vi "CAPTH-Init IPC.vi"() -> (8 "IPC":T1)   [LabVIEW 2020]
uses:
  Typedefs/CAPTH-IPC.ctl
  Typedefs/CAPTH-Start Data.ctl
  Typedefs/CAPTH-Parameters.ctl
  Typedefs/CAPTH-Stimulus.ctl
  Typedefs/CAPTH-Response.ctl
  Typedefs/CAPTH-Analysis Message.ctl
  Typedefs/CAPTH-Analysis Action.ctl
  Typedefs/CAPTH-StimCon.ctl
  Typedefs/CAPTH-Analysis Data Properties.ctl
panel:
  out "queue out":refnum<queue>
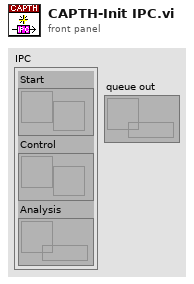
[diagram p1: front panel]
types:
  T1 = typedef "CAPTH-IPC.ctl" = cluster{"Start":refnum<notifier>, "Control":refnum<notifier>, "Analysis":refnum<queue>}
  T2 = typedef "CAPTH-Analysis Message.ctl" = cluster{"Action":T3, "Data":dbl[], "StimCon":T4, "Properties":T5, "Num":i32}
  T3 = typedef "CAPTH-Analysis Action.ctl" = enum16{"Init", "Raw", "Avg", "Quit"}
  T4 = typedef "CAPTH-StimCon.ctl" = cluster{"ear":i32, "freq":i32, "Max SPL":dbl}
  T5 = typedef "CAPTH-Analysis Data Properties.ctl" = cluster{"atten":dbl, "amp":dbl, "1dB":bool}
  T6 = typedef "CAPTH-Start Data.ctl" = cluster{"Datafile":path, "Params":T7, "data":cluster{"Freq":dbl[], "Threshold atten":dbl[], "Max SPL":dbl[]}[]}
  T7 = typedef "CAPTH-Parameters.ctl" = cluster{"Stimulus":T8, "Response":T9}
  T8 = typedef "CAPTH-Stimulus.ctl" = cluster{"EAR":enum16{"RIGHT", "LEFT\n", "ALTERNATE"}, "HI FREQ":dbl, "LO FREQ":dbl, "FREQ STEP":u8, "Rep Rate (/s)":dbl, "Alternate Polarity":bool, "# CYCLES":u8, "Duration (ms)":dbl, "Ramp (ms)":dbl}
  T9 = typedef "CAPTH-Response.ctl" = cluster{"Averages (3dB steps)":i32, "Time Window (ms)":dbl, "dt (us)":dbl, "Grass gain":dbl, "CRITERION (mV)":dbl, "CEILING (dB atten)":dbl, "Use previous":bool, "Save avgs":bool, "Save raw":bool, "Save history":bool, "CEILING (dB SPL)":dbl}
  T10 = cluster{"notifier out":refnum<notifier>, "notifier out":refnum<notifier>, "queue out":refnum<queue>}
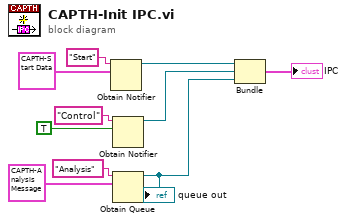
[diagram p0: block diagram]
diagram:
  n1 = Obtain Notifier(name (unnamed)="Start", notification data type=T6 {"Datafile"=path "", "Params"={"Stimulus"={"EAR"=enum."RIGHT", "HI FREQ"=0.0, "LO FREQ"=0.0, "FREQ STEP"=0, "Rep Rate (/s)"=0.0, "Alternate Polarity"=FALSE, "# CYCLES"=0, "Duration (ms)"=0.0, "Ramp (ms)"=0.0}, "Response"={"Averages (3dB steps)"=0, "Time Window (ms)"=0.0, "dt (us)"=0.0, "Grass gain"=0.0, "CRITERION (mV)"=0.0, "CEILING (dB atten)"=0.0, "Use previous"=FALSE, "Save avgs"=FALSE, "Save raw"=FALSE, "Save history"=FALSE, "CEILING (dB SPL)"=6.0}}, "data"=[]} ("Start")) -> (notifier out=w6:refnum<notifier>)  [unwired: 2 in, 2 out]
  n2 = Obtain Notifier(name (unnamed)="Control", notification data type=TRUE) -> (notifier out=w5:refnum<notifier>)  [unwired: 2 in, 2 out]
  n3 = Obtain Queue(name (unnamed)="Analysis", element data type=T2 {"Action"=enum."Init", "Data"=[], "StimCon"={"ear"=0, "freq"=0, "Max SPL"=0.0}, "Properties"={"atten"=0.0, "amp"=0.0, "1dB"=FALSE}, "Num"=0} ("Message")) -> (queue out=w1:refnum<queue>)  [unwired: 3 in, 2 out]
  "queue out" <- w1
  n4 = Bundle("notifier out"=w6, "notifier out"=w5, "queue out"=w1) -> (→"IPC":T10)  [unwired: 1 in]
